vi "1-13.vi"() -> ()   [LabVIEW 2022 SP3]
panel:
  out "最后结果":dbl
  out "相乘的结果":dbl
  out "产生的随机数":dbl
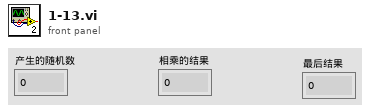
[diagram p1: front panel]
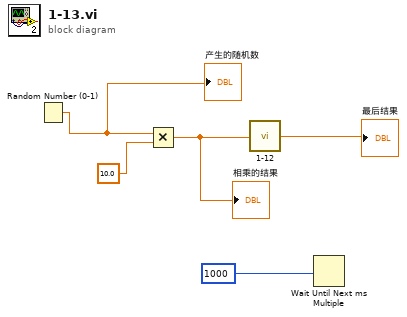
[diagram p0: block diagram]
diagram:
  n1 = Random Number (0-1)() -> (number: 0 to 1=w3:dbl)
  "产生的随机数" <- w3
  n2 = Multiply(x=w3, y=10.0) -> (x*y=w2:dbl)
  "相乘的结果" <- w2
  n3 = call "1-12.vi"("数值 2"=w2) -> ("数值"=→"最后结果":dbl)
  n4 = Wait Until Next ms Multiple(millisecond multiple=1000) -> ()  [unwired: 1 out]
